vi "SubVICreate.vi"(0 "__args":T1) -> (1 "__return":cluster{"UID":i32, i32[]}, 2 "__errStatus":bool, 3 "__errCode":i32, 4 "__errSource":string)   [LabVIEW 2013]
uses:
  <vilib>/Utility/miscctls.llb/LVPointTypeDef.ctl
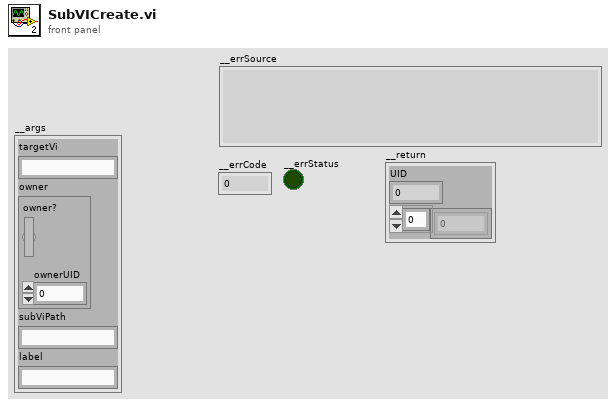
[diagram p1: front panel]
types:
  T1 = cluster{"targetVi":string, "owner":cluster{"owner?":bool, "ownerUID":i32}, "subViPath":string, "label":string}
  T2 = typedef "LVPointTypeDef.ctl" = cluster{"Horizontal":i16, "Vertical":i16}
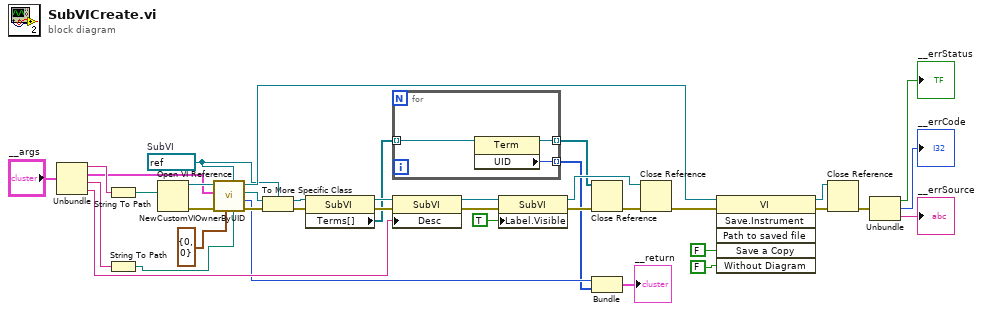
[diagram p0: block diagram]
diagram:
  w11 = refnum<vi> refnum  # SubVI
  n1 = Unbundle("__args") -> ("targetVi"=w14:string, "owner"=w13:cluster{"owner?":bool, "ownerUID":i32}, "subViPath"=w12:string, "label"=w10:string)
  n2 = String To Path(string=w14) -> (path=w38:path)
  n3 = String To Path(string=w12) -> (path=w8:path)
  n4 = Open VI Reference(vi path=w38) -> (vi reference=w22:refnum<vi>, error out=w20:errorcluster)  [unwired: 5 in]
  n5 = call "NewCustomVIOwnerByUID.vi"("path"=w8, "vi object class"=w11, "location"=T2 {"Horizontal"=0, "Vertical"=0}, "error in (no error)"=w20, "owner"=w13, "targetVI"=w22) -> ("error out"=w17:errorcluster, "UID"=w9:i32, "object refnum"=w18:refnum<vi>, "dup targetVI"=w23:refnum<vi>)  [unwired: 2 in]
  n6 = To More Specific Class(target class=w11, reference=w18, error in=w17) -> (specific class reference=w19:refnum<vi>, error out=w16:errorcluster)
  n7 = property class="SubVI"(reference=w19, error in=w16) -> (reference out=w28:refnum<vi>, error out=w27:errorcluster, "Terms[]"=w4:refnum<vi>[])
  n8 = for {
    tunnel: [w40] -> w5 mode=indexing
    tunnel: w4 -> [w41] mode=indexing
    tunnel: [w39] -> w3 mode=indexing
    n9 = property class="Term"(reference=w41) -> (reference out=w40:refnum<vi>, "UID"=w39:i32)  [unwired: 1 in, 1 out]
  }
  n10 = property class="SubVI"(reference=w28, error in=w27, "Desc"=w10) -> (reference out=w26:refnum<vi>, error out=w25:errorcluster)
  n11 = property class="SubVI"(reference=w26, error in=w25, "Label.Visible"=TRUE) -> (reference out=w24:refnum<vi>, error out=w6:errorcluster)
  n12 = Close Reference(reference=w5, error in (no error)=w6) -> (error out=w7:errorcluster)
  n13 = Bundle("UID"=w9, w3) -> (→"__return":cluster{"UID":i32, i32[]})  [unwired: 1 in]
  n14 = Close Reference(reference=w24, error in (no error)=w7) -> (error out=w32:errorcluster)
  n15 = invoke class="VI" method="Save.Instrument"(reference=w23, error in=w32, "Save a Copy"=FALSE, "Without Diagram"=FALSE) -> (reference out=w33:refnum<vi>, error out=w31:errorcluster)  [unwired: 2 in, 4 out]
  n16 = Close Reference(reference=w33, error in (no error)=w31) -> (error out=w34:errorcluster)
  n17 = Unbundle(w34) -> ("status"=→"__errStatus":bool, "code"=→"__errCode":i32, "source"=→"__errSource":string)
